vi "Test Main.vi"() -> ()   [LabVIEW 2020]
uses:
  ExecAnchor/ExecAnchor.lvclass
panel:
  in  "stop":bool
  out "Count":i32
  # "Stop this VI to also stop the async VI."
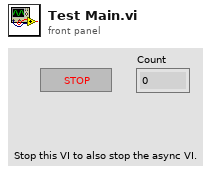
[diagram p1: front panel]
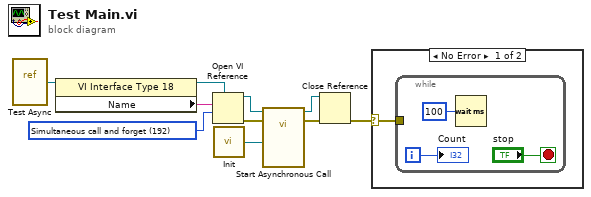
[diagram p0: block diagram]
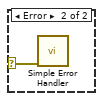
[diagram p2: hidden frame]
diagram:
  w5 = 192 items=["Record modifications"=1, "Open templates for editing"=2, "Prompt user to save"=4, "Prepare for reentrant run"=8, "Prompt to find missing subVIs"=16, "Hide loading dialog box"=32, "Enable simultaneous calls"=64, "Prepare to call and forget"=128, "Simultaneous call and forget"=192, "Prepare to call and collect"=256, "Simultaneous call and collect"=320]
  n1 = vi-ref "Test Async.vi"() -> (w3:refnum<vi>)
  n2 = property class="VI Interface Type 18"(reference=w3) -> (reference out=w6:refnum<vi>, "Name"=w4:string)  [unwired: 1 in, 1 out]
  n3 = Open VI Reference(type specifier VI Refnum (for type only)=w6, vi path=w4, options=w5) -> (vi reference=w8:refnum<vi>, error out=w7:errorcluster)  [unwired: 3 in]
  n4 = call "Init.vi"() -> ("ExecAnchor out"=w2:refnum<class "ExecAnchor.lvclass">)  [unwired: 7 in]
  n5 = call-by-ref "Start Asynchronous Call"(reference=w8, error in=w7, "ExecAnchor"=w2) -> (reference out=w10:refnum<vi>, error out=w9:errorcluster)  [unwired: 11 in]
  n6 = Close Reference(reference=w10, error in (no error)=w9) -> (error out=w1:errorcluster)
  n7 = case shown="No Error" w1 {
    selector: w1 -> [w11 w15]
    frame No Error {
      n8 = while {
        tunnel: w11 -> [_]
        i -> [w14]
        stop <- "stop" stop-if-true
        n9 = Wait (ms)(milliseconds to wait=u32 100) -> ()  [unwired: 1 out]
        "Count" <- w14
      }
    }
    frame Error {
      n10 = call <vilib>:"Simple Error Handler.vi"("error in (no error)"=w15) -> ()  [unwired: 4 in, 5 out]
    }
  }
